vi "BuildTwoLineString.vi"(9 "SecondLineString":string, 11 "FirstLineString":string) -> (2 "TwoLineString":string)   [LabVIEW 2021]
doc: "jiangsong:\njiangsong@outlook.com\n\n20140426"
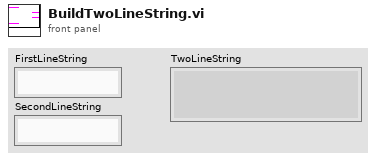
[diagram p1: front panel]
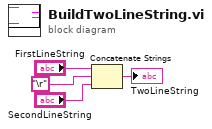
[diagram p0: block diagram]
diagram:
  n1 = Concatenate Strings("FirstLineString", "\r", "SecondLineString") -> (→"TwoLineString":string)
